vi "Servo Close.vi"   [LabVIEW 2011, in "LMH-LINX.lvlib" / "Servo.lvlib"]
uses:
  Servo.lvlib
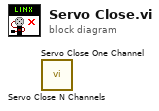
[diagram p0: block diagram]
diagram:
  n1 = call "Servo Close N Channels.vi"() -> ()  [unwired: 10 in, 2 out]
  n2 = call "Servo Close One Channel.vi"() -> ()  [unwired: 10 in, 2 out]
